vi "Auto Drive.vi"(0 "Ticks(Distance)":dbl=2445.0 format="%#_13g", 1 "Swerve DevRef":T2[](array[typedef])=[{"DeviceStatus"={"status"=FALSE, "code"=0, "source"=""}, "Type"=enum."CAN", "PWM"={"PWM Channel"=enum."PWM 1", "DeadBand"={"Name"="", "maxPositivePwm"=0, "minPositivePwm"=0, "centerPwm"=0, "maxNegativePwm"=0, "minNegativePwm"=0, "angularRange"=0}}, "CAN"={"Device Number"=4, "SetOutput VI Ref"=variant(refnum<vi> refnum), "GetOutput VI Ref"=variant(refnum<vi> refnum), "Enable VI Ref"=variant(refnum<vi> refnum), "Disable VI Ref"=variant(refnum<vi> refnum), "Data"=variant(cluster{"Control Mode":enum8{"Percent VBus", "Speed", "Position", "Slave", "Unchanged / Invalid", "Voltage Compensation", "Current", "Motion Profile", "Motion Magic"}, "Encoder Initial Position":dbl, "MaxVout":dbl} {"Control Mode"=enum."Position", "Encoder Initial Position"=0.0, "MaxVout"=12.0})}, "Invert"=FALSE}, {"DeviceStatus"={"status"=FALSE, "code"=0, "source"=""}, "Type"=enum."CAN", "PWM"={"PWM Channel"=enum."PWM 1", "DeadBand"={"Name"="", "maxPositivePwm"=0, "minPositivePwm"=0, "centerPwm"=0, "maxNegativePwm"=0, "minNegativePwm"=0, "angularRange"=0}}, "CAN"={"Device Number"=8, "SetOutput VI Ref"=variant(refnum<vi> refnum), "GetOutput VI Ref"=variant(refnum<vi> refnum), "Enable VI Ref"=variant(refnum<vi> refnum), "Disable VI Ref"=variant(refnum<vi> refnum), "Data"=variant(cluster{"Control Mode":enum8{"Percent VBus", "Speed", "Position", "Slave", "Unchanged / Invalid", "Voltage Compensation", "Current", "Motion Profile", "Motion Magic"}, "Encoder Initial Position":dbl, "MaxVout":dbl} {"Control Mode"=enum."Position", "Encoder Initial Position"=0.0, "MaxVout"=12.0})}, "Invert"=FALSE}, {"DeviceStatus"={"status"=FALSE, "code"=0, "source"=""}, "Type"=enum."CAN", "PWM"={"PWM Channel"=enum."PWM 1", "DeadBand"={"Name"="", "maxPositivePwm"=0, "minPositivePwm"=0, "centerPwm"=0, "maxNegativePwm"=0, "minNegativePwm"=0, "angularRange"=0}}, "CAN"={"Device Number"=6, "SetOutput VI Ref"=variant(refnum<vi> refnum), "GetOutput VI Ref"=variant(refnum<vi> refnum), "Enable VI Ref"=variant(refnum<vi> refnum), "Disable VI Ref"=variant(refnum<vi> refnum), "Data"=variant(cluster{"Control Mode":enum8{"Percent VBus", "Speed", "Position", "Slave", "Unchanged / Invalid", "Voltage Compensation", "Current", "Motion Profile", "Motion Magic"}, "Encoder Initial Position":dbl, "MaxVout":dbl} {"Control Mode"=enum."Position", "Encoder Initial Position"=0.0, "MaxVout"=12.0})}, "Invert"=FALSE}, {"DeviceStatus"={"status"=FALSE, "code"=0, "source"=""}, "Type"=enum."CAN", "PWM"={"PWM Channel"=enum."PWM 1", "DeadBand"={"Name"="", "maxPositivePwm"=0, "minPositivePwm"=0, "centerPwm"=0, "maxNegativePwm"=0, "minNegativePwm"=0, "angularRange"=0}}, "CAN"={"Device Number"=2, "SetOutput VI Ref"=variant(refnum<vi> refnum), "GetOutput VI Ref"=variant(refnum<vi> refnum), "Enable VI Ref"=variant(refnum<vi> refnum), "Disable VI Ref"=variant(refnum<vi> refnum), "Data"=variant(cluster{"Control Mode":enum8{"Percent VBus", "Speed", "Position", "Slave", "Unchanged / Invalid", "Voltage Compensation", "Current", "Motion Profile", "Motion Magic"}, "Encoder Initial Position":dbl, "MaxVout":dbl} {"Control Mode"=enum."Position", "Encoder Initial Position"=0.0, "MaxVout"=12.0})}, "Invert"=FALSE}], 5 "Drive Angle":dbl=3.141592653589793, 7 "Start Power":dbl=0.2 format="%#_13g", 9 "Time Condition":u32=10000, 11 "error in":errorcluster={"status"=FALSE, "code"=44087, "source"="NetComm_CAN_Send.vi:5830003<APPEND>\n\n<b>Complete call chain:</b>\n     NetComm_CAN_Send.vi:5830003\n     WPI_CANTalonSRX_Send.vi\n     WPI_CANTalonSRX_SetOutput.vi\n     WPI_MotorControlSetOutput.vi\n     Drive Direction.vi:1350004\n     Drive.vi:820003\n     Auto Drive.vi\n     Place Front Gear.vi\n     Autonomous Independent.vi"}, 12 "Wheel DevRef":T2[](array[typedef])=[{"DeviceStatus"={"status"=FALSE, "code"=0, "source"=""}, "Type"=enum."CAN", "PWM"={"PWM Channel"=enum."PWM 1", "DeadBand"={"Name"="", "maxPositivePwm"=0, "minPositivePwm"=0, "centerPwm"=0, "maxNegativePwm"=0, "minNegativePwm"=0, "angularRange"=0}}, "CAN"={"Device Number"=3, "SetOutput VI Ref"=variant(refnum<vi> refnum), "GetOutput VI Ref"=variant(refnum<vi> refnum), "Enable VI Ref"=variant(refnum<vi> refnum), "Disable VI Ref"=variant(refnum<vi> refnum), "Data"=variant(cluster{"Control Mode":enum8{"Percent VBus", "Speed", "Position", "Slave", "Unchanged / Invalid", "Voltage Compensation", "Current", "Motion Profile", "Motion Magic"}, "Encoder Initial Position":dbl, "MaxVout":dbl} {"Control Mode"=enum."Percent VBus", "Encoder Initial Position"=0.0, "MaxVout"=12.0})}, "Invert"=TRUE}, {"DeviceStatus"={"status"=FALSE, "code"=0, "source"=""}, "Type"=enum."CAN", "PWM"={"PWM Channel"=enum."PWM 1", "DeadBand"={"Name"="", "maxPositivePwm"=0, "minPositivePwm"=0, "centerPwm"=0, "maxNegativePwm"=0, "minNegativePwm"=0, "angularRange"=0}}, "CAN"={"Device Number"=7, "SetOutput VI Ref"=variant(refnum<vi> refnum), "GetOutput VI Ref"=variant(refnum<vi> refnum), "Enable VI Ref"=variant(refnum<vi> refnum), "Disable VI Ref"=variant(refnum<vi> refnum), "Data"=variant(cluster{"Control Mode":enum8{"Percent VBus", "Speed", "Position", "Slave", "Unchanged / Invalid", "Voltage Compensation", "Current", "Motion Profile", "Motion Magic"}, "Encoder Initial Position":dbl, "MaxVout":dbl} {"Control Mode"=enum."Percent VBus", "Encoder Initial Position"=0.0, "MaxVout"=12.0})}, "Invert"=TRUE}, {"DeviceStatus"={"status"=FALSE, "code"=0, "source"=""}, "Type"=enum."CAN", "PWM"={"PWM Channel"=enum."PWM 1", "DeadBand"={"Name"="", "maxPositivePwm"=0, "minPositivePwm"=0, "centerPwm"=0, "maxNegativePwm"=0, "minNegativePwm"=0, "angularRange"=0}}, "CAN"={"Device Number"=5, "SetOutput VI Ref"=variant(refnum<vi> refnum), "GetOutput VI Ref"=variant(refnum<vi> refnum), "Enable VI Ref"=variant(refnum<vi> refnum), "Disable VI Ref"=variant(refnum<vi> refnum), "Data"=variant(cluster{"Control Mode":enum8{"Percent VBus", "Speed", "Position", "Slave", "Unchanged / Invalid", "Voltage Compensation", "Current", "Motion Profile", "Motion Magic"}, "Encoder Initial Position":dbl, "MaxVout":dbl} {"Control Mode"=enum."Percent VBus", "Encoder Initial Position"=0.0, "MaxVout"=12.0})}, "Invert"=FALSE}, {"DeviceStatus"={"status"=FALSE, "code"=0, "source"=""}, "Type"=enum."CAN", "PWM"={"PWM Channel"=enum."PWM 1", "DeadBand"={"Name"="", "maxPositivePwm"=0, "minPositivePwm"=0, "centerPwm"=0, "maxNegativePwm"=0, "minNegativePwm"=0, "angularRange"=0}}, "CAN"={"Device Number"=1, "SetOutput VI Ref"=variant(refnum<vi> refnum), "GetOutput VI Ref"=variant(refnum<vi> refnum), "Enable VI Ref"=variant(refnum<vi> refnum), "Disable VI Ref"=variant(refnum<vi> refnum), "Data"=variant(cluster{"Control Mode":enum8{"Percent VBus", "Speed", "Position", "Slave", "Unchanged / Invalid", "Voltage Compensation", "Current", "Motion Profile", "Motion Magic"}, "Encoder Initial Position":dbl, "MaxVout":dbl} {"Control Mode"=enum."Percent VBus", "Encoder Initial Position"=0.0, "MaxVout"=12.0})}, "Invert"=FALSE}]) -> (15 "error out":errorcluster)   [LabVIEW 2016]
uses:
  <vilib>/Rock Robotics/WPI/MotorControl/WPI_MotorControlDeviceRef.ctl
  <vilib>/Rock Robotics/WPI/MotorControl/WPI_MotorControlType.ctl
  <vilib>/Rock Robotics/SystemInterfaces/DIO/FPGA_DIOPWMChannel.ctl
  <vilib>/Rock Robotics/WPI/PWM/WPI_PWMDeadband.ctl
  <vilib>/addons/control/pid/pid.llb/PID (DBL).vi
  <vilib>/addons/control/pid/NI_PID_pid.lvlib
panel:
  out "Wheel Speed Waveform":cluster{"Wheel Speed":dbl}[](graph)
  out "Wheel 1":dbl(graph)=0.7087321764785622
  out "Wheel 3 Chart":dbl(graph)=0.7087321764785622
  out "Z":dbl(graph)=-1.0
  out "Difference":dbl(graph)=6835.0
  in  "output range":cluster{"output high":dbl, "output low":dbl}={"output high"=1.0, "output low"=-1.0} {"output low" format="%.2f"; "output high" format="%.2f"}
  in  "PID gains Rotational Correction":T1={"proportional gain (Kc)"=2.5e-05, "integral time (Ti, min)"=0.0, "derivative time (Td, min)"=0.0} {"derivative time (Td, min)" format="%.3f"; "integral time (Ti, min)" format="%.3f"; "proportional gain (Kc)" format="%.9f"}
  # ".000025"
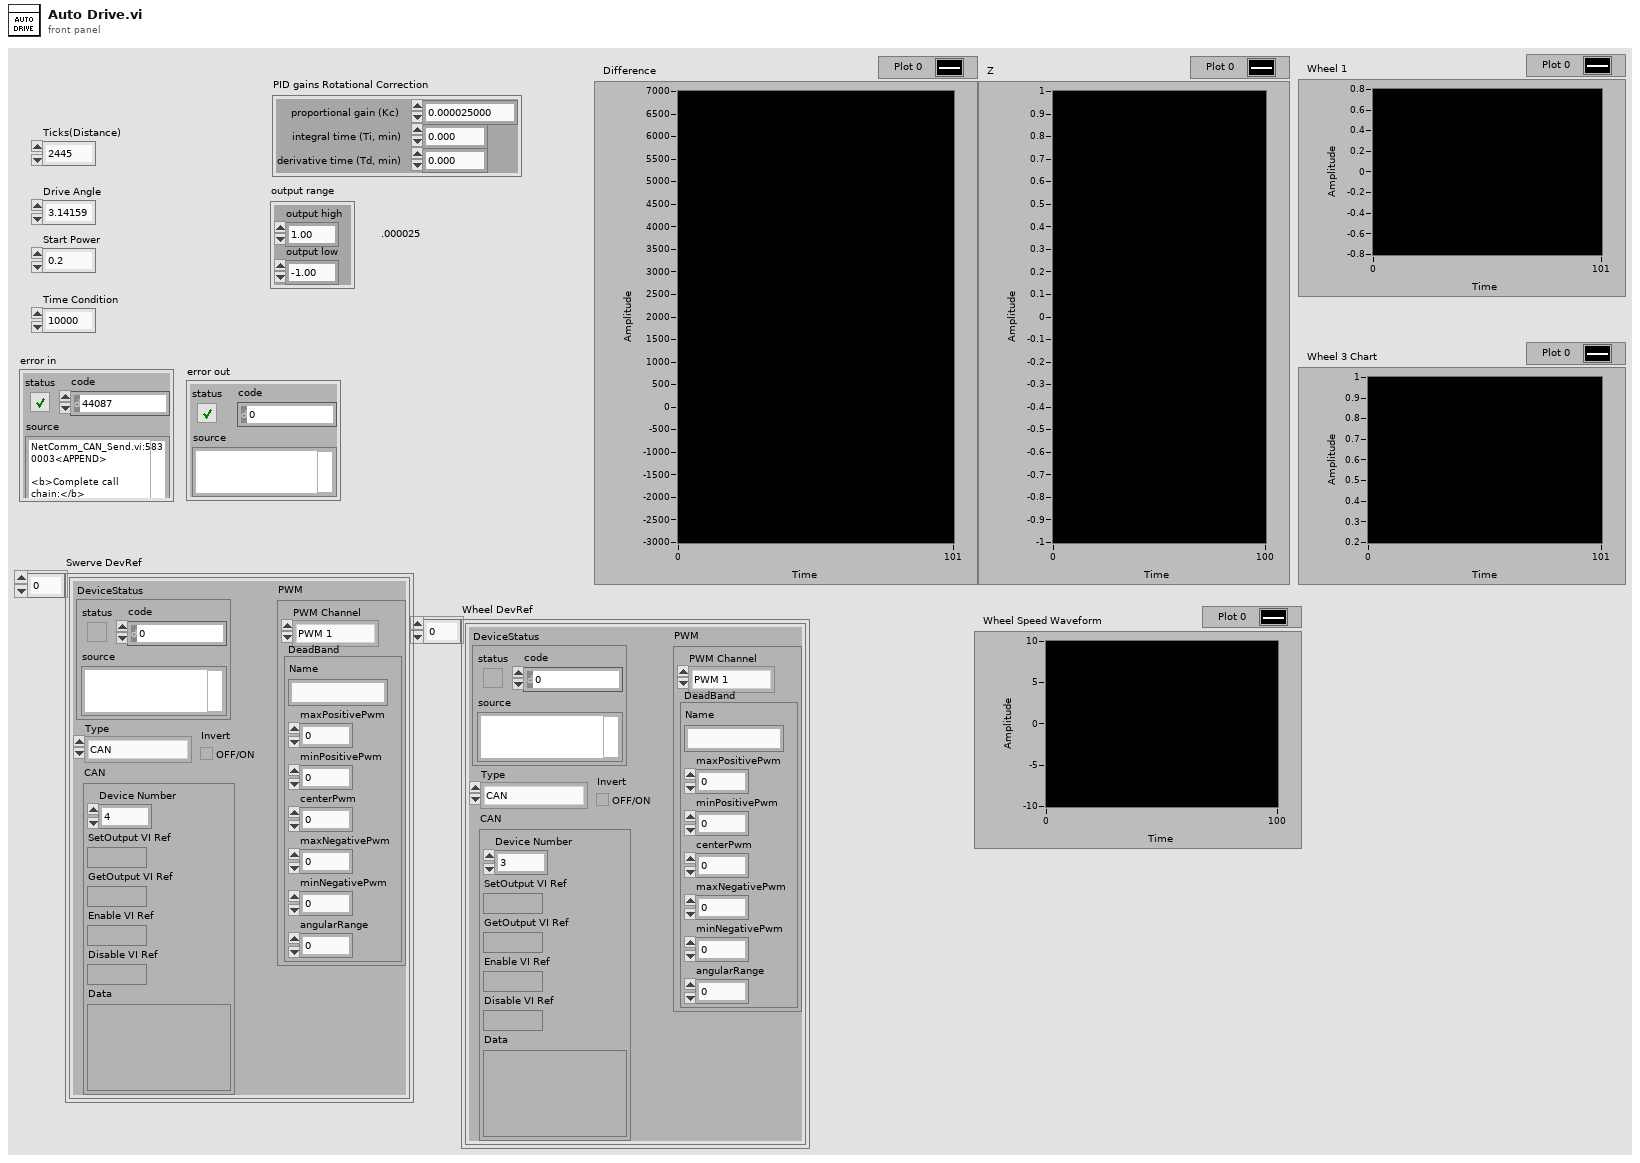
[diagram p1: front panel]
types:
  T1 = cluster{"proportional gain (Kc)":dbl, "integral time (Ti, min)":dbl, "derivative time (Td, min)":dbl}
  T2 = typedef "WPI_MotorControlDeviceRef.ctl" = cluster{"DeviceStatus":errorcluster, "Type":T3, "PWM":cluster{"PWM Channel":T4, "DeadBand":T5}, "CAN":cluster{"Device Number":u8, "SetOutput VI Ref":variant, "GetOutput VI Ref":variant, "Enable VI Ref":variant, "Disable VI Ref":variant, "Data":variant}, "Invert":bool}
  T3 = typedef "WPI_MotorControlType.ctl" = enum16{"PWM", "CAN"}
  T4 = typedef "FPGA_DIOPWMChannel.ctl" = enum8{"PWM 0", "PWM 1", "PWM 2", "PWM 3", "PWM 4", "PWM 5", "PWM 6", "PWM 7", "PWM 8", "PWM 9", "PWM MXP 0", "PWM MXP 1", "PWM MXP 2", "PWM MXP 3", "PWM MXP 4", "PWM MXP 5", "PWM MXP 6", "PWM MXP 7", "PWM MXP 8", "PWM MXP 9", "Invalid"}
  T5 = typedef "WPI_PWMDeadband.ctl" = cluster{"Name":string, "maxPositivePwm":i32, "minPositivePwm":i32, "centerPwm":i32, "maxNegativePwm":i32, "minNegativePwm":i32, "angularRange":u16}
  T6 = typedef "WPI_CANTalonSRX_GlobalStatus.ctl" = cluster{"Applied Throttle":dbl, "Module Enabled":bool, "CAN Error":errorcluster, "Closed Loop Error":dbl, "Forward Limit Switch Closed":bool, "Reverse Limit Switch Closed":bool, "Sensor Position":dbl, "Sensor Velocity":dbl, "Current":dbl, "Sticky Fault - Over Temp":bool, "Sticky Fault - Under Voltage":bool, "Sticky Fault - Forward Limit":bool, "Sticky Fault - Reverse Limit":bool, "Sticky Fault - Forward Soft Limit":bool, "Sticky Fault - Reverse Soft Limit":bool, "Brake is Enabled":bool, "Encoder Position":dbl, "Encoder Velocity":dbl, "Encoder Index Count":dbl, "Encoder A Pin State":bool, "Encoder B Pin State":bool, "Encoder Index Pin State":bool, "Analog In":dbl, "Analog In Velocity":dbl, "Temperature (C)":dbl, "Battery Voltage":dbl, "Control 5 Is Supported":bool, "Current Profile Slot Select":dbl, "Pos Div 8":bool, "Vel Div 4":bool, "Pulse Width Position":i32, "Pulse Width Velocity":i32, "Pulse Width Rise To Rise (us)":i32, "Pulse Width Rise To Fall (us)":i32, "Mot Prof Active Is Under Run":bool, "Mot Prof Active Has Under Run":bool, "Mot Prof Active Is Last":bool, "Mot Prof Active Velocity Only":bool, "Mot Prof Active Is Valid":bool, "Mot Prof Buffer Is Full":bool, "Mot Prof Active Profile Slot Select":i32, "Mot Prof NextID":i32, "Mot Prof Count":i32, "Mot Prof Active Velocity":dbl, "Mot Prof Active Position":dbl, "Mot Prof Output Enable":i32}
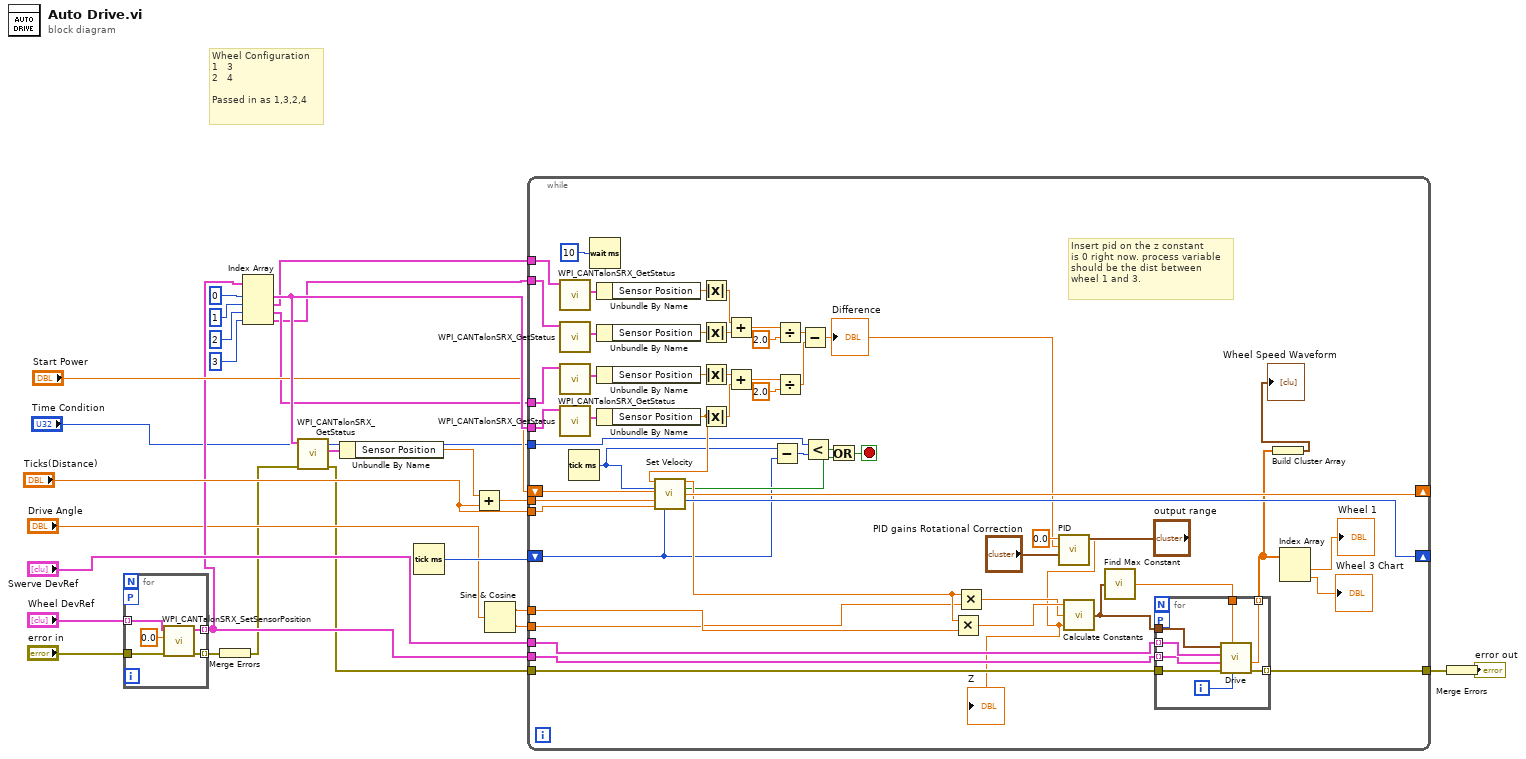
[diagram p0: block diagram]
diagram:
  # "Wheel Configuration\n1   3\n2   4\n\nPassed in as 1,3,2,4"
  n1 = for {
    tunnel: "Wheel DevRef" -> [w32] mode=indexing
    tunnel: [w30] -> w16 mode=indexing
    workers-P: _ -> [_]
    tunnel: "error in" -> [w29]
    tunnel: [w28] -> w8 mode=indexing
    n2 = call <vilib>:"WPI_CANTalonSRX_SetSensorPosition.vi"("error in (no error)"=w29, "New Sensor Position"=0.0, "CAN Talon SRX Ref"=w32) -> ("error out"=w28:errorcluster, "CAN Talon SRX Ref"=w30:T2)  [unwired: 7 in]
  }
  n3 = Merge Errors(w8) -> (w7:errorcluster)
  n4 = Index Array(array=w16, index #1=0 ("index"), index #2=1 ("index"), index #3=2 ("index"), index #4=3 ("index")) -> (element #1=w22:T2, element #2=w10:T2, element #3=w3:T2, element #4=w2:T2)
  n5 = call <vilib>:"WPI_CANTalonSRX_GetStatus.vi"("error in (no error)"=w7, "CAN Talon SRX Ref"=w22) -> ("error out"=w6:errorcluster, "Talon SRX Status"=w26:T6)  [unwired: 7 in, 1 out]
  n6 = Unbundle By Name(w26) -> ("Sensor Position"=w24:dbl)
  n7 = Tick Count (ms)() -> (millisecond timer value=w18:u32)
  n8 = Add(x=w24, y="Ticks(Distance)") -> (x+y=w23:dbl)
  n9 = Sine & Cosine(0:"Drive Angle") -> (1:w15:dbl, 2:w14:dbl)
  n10 = while {
    tunnel: w6 -> [w81]
    tunnel: [w82] -> w20
    tunnel: "Swerve DevRef" -> [w87]
    tunnel: w23 -> [w84]
    tunnel: w16 -> [w86]
    tunnel: w22 -> [w85]
    tunnel: "Ticks(Distance)" -> [w83]
    shift-right: [w79] -> _
    shift-left: "Start Power" -> [w80]
    shift-right: [w78] -> _
    shift-left: w18 -> [w33]
    tunnel: w15 -> [w72]
    tunnel: w14 -> [w71]
    tunnel: w10 -> [w69]
    tunnel: w3 -> [w57]
    tunnel: w2 -> [w51]
    tunnel: "Time Condition" -> [w38]
    stop <- w37 stop-if-true
    # "Insert pid on the z constant\nis 0 right now. process variable\nshould be the dist between \nwheel 1 and 3."
    n11 = call <vilib>:"WPI_CANTalonSRX_GetStatus.vi"("CAN Talon SRX Ref"=w69) -> ("Talon SRX Status"=w70:T6)  [unwired: 8 in, 2 out]
    n12 = call <vilib>:"WPI_CANTalonSRX_GetStatus.vi"("CAN Talon SRX Ref"=w51) -> ("Talon SRX Status"=w50:T6)  [unwired: 8 in, 2 out]
    n13 = call <vilib>:"WPI_CANTalonSRX_GetStatus.vi"("CAN Talon SRX Ref"=w57) -> ("Talon SRX Status"=w58:T6)  [unwired: 8 in, 2 out]
    n14 = call <vilib>:"WPI_CANTalonSRX_GetStatus.vi"("CAN Talon SRX Ref"=w85) -> ("Talon SRX Status"=w76:T6)  [unwired: 8 in, 2 out]
    n15 = Tick Count (ms)() -> (millisecond timer value=w34:u32)
    n16 = Wait (ms)(milliseconds to wait=u32 10) -> ()  [unwired: 1 out]
    n17 = Unbundle By Name(w70) -> ("Sensor Position"=w68:dbl)
    n18 = Unbundle By Name(w50) -> ("Sensor Position"=w52:dbl)
    n19 = Unbundle By Name(w58) -> ("Sensor Position"=w56:dbl)
    n20 = Unbundle By Name(w76) -> ("Sensor Position"=w67:dbl)
    n21 = call "Set Velocity.vi"("Process Variable(x)"=w67, "Current TIme"=w34, "Current Power"=w80, "Setpoint(end)"=w84, "Total Distance"=w83, "Last Time Input"=w33) -> ("Coerced Motor power"=w77:dbl, "End Loop?"=w42:bool, "Non-Coerced Motor Power"=w79:dbl, "Last Time Output"=w78:u32)  [unwired: 6 in]
    n22 = Absolute Value(x=w68) -> (abs(x)=w48:dbl)
    n23 = Absolute Value(x=w52) -> (abs(x)=w49:dbl)
    n24 = Absolute Value(x=w56) -> (abs(x)=w54:dbl)
    n25 = Absolute Value(x=w67) -> (abs(x)=w53:dbl)
    n26 = Add(x=w48, y=w49) -> (x+y=w47:dbl)
    n27 = Add(x=w54, y=w53) -> (x+y=w55:dbl)
    n28 = Subtract(x=w34, y=w33) -> (x-y=w35:u32)
    n29 = Divide(x=w47, y=2.0) -> (x/y=w43:dbl)
    n30 = Divide(x=w55, y=2.0) -> (x/y=w44:dbl)
    n31 = Subtract(x=w43, y=w44) -> (x-y=w41:dbl)
    "Difference" <- w41
    n32 = Less?(x=w38, y=w35) -> (x < y?=w36:bool)
    n33 = Or(x=w36, y=w42) -> (x .or. y?=w37:bool)
    n34 = Multiply(x=w77, y=w72) -> (x*y=w75:dbl)
    n35 = Multiply(x=w77, y=w71) -> (x*y=w74:dbl)
    n36 = call-poly <vilib>:"PID.vi"("output range"="output range", "PID gains"="PID gains Rotational Correction", "process variable"=w41, "setpoint"=0.0) -> ("output"=w61:dbl)  [unwired: 6 in, 1 out]
    "Z" <- w61
    n37 = call "Calculate Constants.vi"("Z"=w61, "Y"=w74, "X"=w75) -> ("constants cluster"=w62:cluster{"a":dbl, "b":dbl, "c":dbl, "d":dbl})
    n38 = call "Find Max Constant.vi"("constants"=w62) -> ("Max or 1"=w63:dbl)
    n39 = for {
      tunnel: w62 -> [w95]
      tunnel: w87 -> [w94] mode=indexing
      tunnel: w86 -> [w93] mode=indexing
      workers-P: _ -> [_]
      tunnel: [w91] -> w82 mode=indexing
      tunnel: w81 -> [w90]
      tunnel: w63 -> [w89]
      tunnel: [w88] -> w40 mode=indexing
      i -> [w92]
      n40 = call "Drive.vi"("Index"=w92, "Max Speed or 1"=w89, "error in"=w90, "Wheel DevRef"=w93, "Swerve DevRef"=w94, "constants"=w95) -> ("error out"=w91:errorcluster, "Wheel Speed"=w88:dbl)  [unwired: 1 in, 3 out]
    }
    n41 = Build Cluster Array(w40) -> (→"Wheel Speed Waveform":cluster{"Wheel Speed":dbl}[])
    n42 = Index Array(array=w40) -> (element #1=→"Wheel 1":dbl, element #2=→"Wheel 3 Chart":dbl)  [unwired: 2 in]
  }
  n43 = Merge Errors(w20) -> (→"error out":errorcluster)
